vi "OpenFile.vi"(2 "error in (no error)":errorcluster, 3 "Filepath":path, 4 "Extra headers":string) -> (0 "error out":errorcluster, 1 "File handle":refnum<file>)   [LabVIEW 2015]
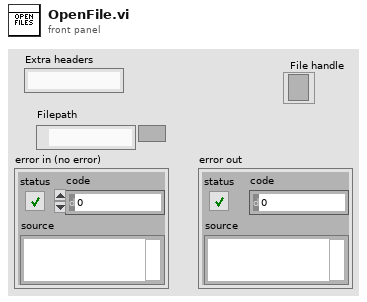
[diagram p1: front panel]
types:
  T1 = enum16{"open", "replace", "create", "open or create", "replace or create", "replace or create with confirmation"}
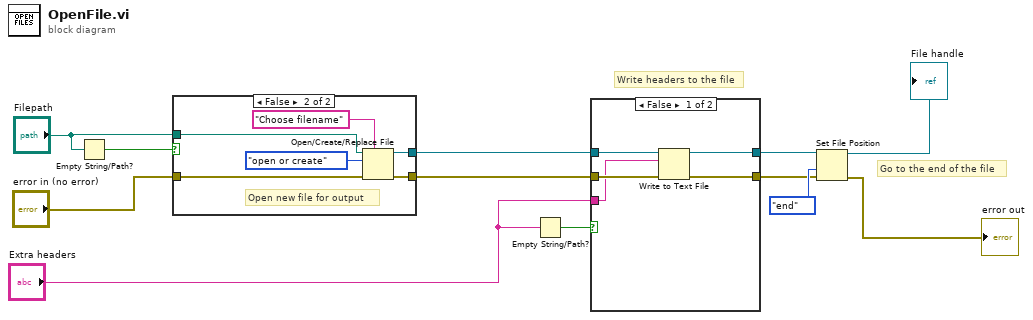
[diagram p0: block diagram]
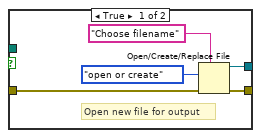
[diagram p3: hidden frame]
diagram:
  # "Go to the end of the file"
  # "Write headers to the file"
  n1 = Empty String/Path?(string/path="Filepath") -> (empty?=w8:bool)
  n2 = case shown="False" w8 {
    tunnel: [w17 w23] -> w2
    tunnel: "error in (no error)" -> [w16 w22]
    tunnel: [w15 w21] -> w1
    tunnel: "Filepath" -> [_ w18]
    frame True {
      # "Open new file for output"
      n3 = Open/Create/Replace File(error in=w16, prompt="Choose filename", operation (0:open)=T1."open or create") -> (refnum out=w15:refnum<file>, error out=w17:errorcluster)  [unwired: 3 in, 1 out]
    }
    frame False {
      # "Open new file for output"
      n4 = Open/Create/Replace File(file path (use dialog)=w18, error in=w22, prompt="Choose filename", operation (0:open)=T1."open or create") -> (refnum out=w21:refnum<file>, error out=w23:errorcluster)  [unwired: 2 in, 1 out]
    }
  }
  n5 = Empty String/Path?(string/path="Extra headers") -> (empty?=w3:bool)
  n6 = case shown="False" w3 {
    tunnel: [w28 w30] -> w6
    tunnel: [w27 w29] -> w5
    tunnel: "Extra headers" -> [w24 _]
    tunnel: w2 -> [w26 w29]
    tunnel: w1 -> [w25 w30]
    frame False {
      n7 = Write to Text File(file (use dialog)=w25, text=w24, error in=w26) -> (refnum out=w28:refnum<file>, error out=w27:errorcluster)  [unwired: 1 in, 1 out]
    }
    frame True {
      # "No headers"
    }
  }
  n8 = Set File Position(refnum=w6, from (0:start)=enum16{"start", "end", "current"}."end", error in=w5) -> (refnum out=→"File handle":refnum<file>, error out=→"error out":errorcluster)  [unwired: 1 in]
